vi "Write State.vi"(8 "error in (no error)":errorcluster, 10 "OpMode":T1=enum."Off", 11 "Lamp Container in":refnum<class "Lamp Container.lvclass">) -> (0 "error out":errorcluster, 3 "Lamp Container out":refnum<class "Lamp Container.lvclass">)   [LabVIEW 2016, in "Lamp Container.lvclass"]
uses:
  Lamp Container.lvclass
  Controls/Operational Modes.ctl
  Lamp Container.lvclass/Lamp Container.ctl
  ThAr/ThAr.lvclass
  LED/LED.lvclass
  Quartz/Quartz.lvclass
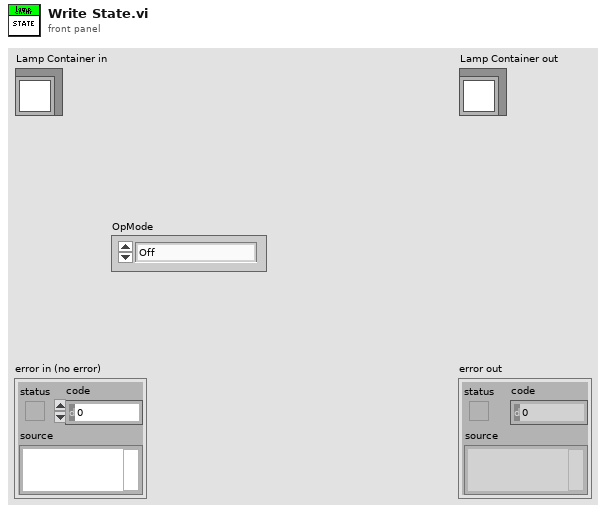
[diagram p1: front panel]
types:
  T1 = typedef "Operational Modes.ctl" = enum16{"Sci", "Sci-LFC", "Solar", "Solar-LFC", "LFC", "LFC-Sim", "LFC-Both", "ThAr", "ThAr-LFC", "Flat", "ExtFlat", "ExtFlat-Sim", "ExtFlat-Both", "Qtz", "ExtQtz", "ExtQtz-Sim", "ExtQtz-Both", "Dark", "Manual", "Off"}
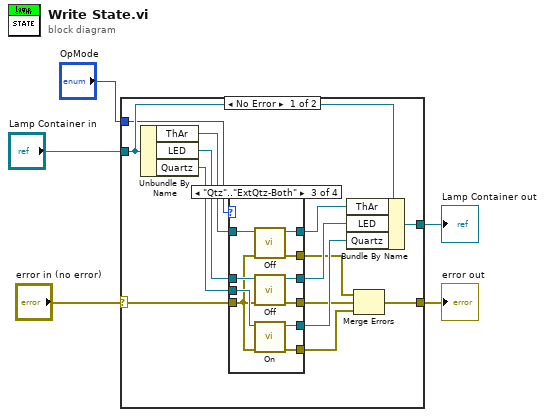
[diagram p0: block diagram]
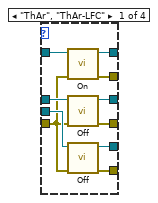
[diagram p2: hidden frame]
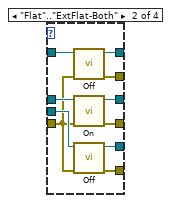
[diagram p3: hidden frame]
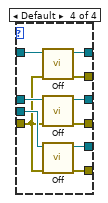
[diagram p4: hidden frame]
diagram:
  n1 = case shown="No Error" "error in (no error)" {
    selector: "error in (no error)" -> [w10 w61]
    tunnel: [w6 w61] -> w4
    tunnel: [w19 w60] -> w2
    tunnel: "Lamp Container in" -> [w18 w60]
    tunnel: "OpMode" -> [w17 _]
    frame No Error {
      n2 = Unbundle By Name(w18) -> ("ThAr"=w16:refnum<class "ThAr.lvclass">, "LED"=w15:refnum<class "LED.lvclass">, "Quartz"=w14:refnum<class "Quartz.lvclass">)
      n3 = case shown="\"Qtz\"..\"ExtQtz-Both\"" w17 {
        tunnel: w16 -> [w23 w39 w46 w59]
        tunnel: w15 -> [w26 w38 w47 w58]
        tunnel: w14 -> [w29 w37 w45 w57]
        tunnel: [w24 w34 w49 w56] -> w13
        tunnel: [w25 w35 w48 w55] -> w12
        tunnel: [w28 w36 w44 w54] -> w11
        tunnel: w10 -> [w22 w30 w40 w53]
        tunnel: [w21 w33 w41 w52] -> w9
        tunnel: [w20 w32 w42 w51] -> w8
        tunnel: [w27 w31 w43 w50] -> w7
        frame "ThAr", "ThAr-LFC" {
          n4 = call-dynamic "On.vi"("error in (no error)"=w22, "ThAr in"=w23) -> ("error out"=w21:errorcluster, "ThAr out"=w24:refnum<class "ThAr.lvclass">)  [unwired: 8 in]
          n5 = call-dynamic "Off.vi"("error in (no error)"=w22, "Lamp in"=w26) -> ("error out"=w20:errorcluster, "Lamp out"=w25:refnum<class "LED.lvclass">)  [unwired: 8 in]
          n6 = call-dynamic "Off.vi"("error in (no error)"=w22, "Lamp in"=w29) -> ("error out"=w27:errorcluster, "Lamp out"=w28:refnum<class "Quartz.lvclass">)  [unwired: 8 in]
        }
        frame "Flat".."ExtFlat-Both" {
          n7 = call-dynamic "Off.vi"("error in (no error)"=w30, "ThAr in"=w39) -> ("error out"=w33:errorcluster, "ThAr out"=w34:refnum<class "ThAr.lvclass">)  [unwired: 8 in]
          n8 = call-dynamic "On.vi"("error in (no error)"=w30, "Lamp in"=w38) -> ("error out"=w32:errorcluster, "Lamp out"=w35:refnum<class "LED.lvclass">)  [unwired: 8 in]
          n9 = call-dynamic "Off.vi"("error in (no error)"=w30, "Lamp in"=w37) -> ("error out"=w31:errorcluster, "Lamp out"=w36:refnum<class "Quartz.lvclass">)  [unwired: 8 in]
        }
        frame "Qtz".."ExtQtz-Both" {
          n10 = call-dynamic "Off.vi"("error in (no error)"=w40, "ThAr in"=w46) -> ("error out"=w41:errorcluster, "ThAr out"=w49:refnum<class "ThAr.lvclass">)  [unwired: 8 in]
          n11 = call-dynamic "Off.vi"("error in (no error)"=w40, "Lamp in"=w47) -> ("error out"=w42:errorcluster, "Lamp out"=w48:refnum<class "LED.lvclass">)  [unwired: 8 in]
          n12 = call-dynamic "On.vi"("error in (no error)"=w40, "Lamp in"=w45) -> ("error out"=w43:errorcluster, "Lamp out"=w44:refnum<class "Quartz.lvclass">)  [unwired: 8 in]
        }
        frame Default {
          n13 = call-dynamic "Off.vi"("error in (no error)"=w53, "ThAr in"=w59) -> ("error out"=w52:errorcluster, "ThAr out"=w56:refnum<class "ThAr.lvclass">)  [unwired: 8 in]
          n14 = call-dynamic "Off.vi"("error in (no error)"=w53, "Lamp in"=w58) -> ("error out"=w51:errorcluster, "Lamp out"=w55:refnum<class "LED.lvclass">)  [unwired: 8 in]
          n15 = call-dynamic "Off.vi"("error in (no error)"=w53, "Lamp in"=w57) -> ("error out"=w50:errorcluster, "Lamp out"=w54:refnum<class "Quartz.lvclass">)  [unwired: 8 in]
        }
      }
      n16 = Bundle By Name(cluster=w18, "ThAr"=w13, "LED"=w12, "Quartz"=w11) -> (w19:refnum<class "Lamp Container.lvclass">)
      n17 = Merge Errors(w9, w8, w7) -> (w6:errorcluster)
    }
    frame Error {
    }
  }
  "error out" <- w4
  "Lamp Container out" <- w2
